vi "PowerSuppliesVoltageControl.vi"(4 "Z+":dbl, 6 "Z-":dbl, 7 "OnOff":bool, 8 "Y+":dbl, 9 "Y-":dbl, 10 "X+":dbl, 11 "X-":dbl) -> (0 "Iz-":dbl)   [LabVIEW 2017]
uses:
  <vilib>/imath/engines/lvmath2/RunTimeEngine/Managers/WorkSpace/UID Generator.vi
  <vilib>/imath/engines/lvmath2/RunTimeEngine/RunTimeType/NIMS_RunTimeType_From StrictType (excl LVString).vi
  <instcachedir>/0/NIMS_RunTimeType_From StrictType (excl LVString)_1019F277F0A747EDBCA0F6C52CA54500.lvgen/NIMS_RunTimeType_From StrictType (excl LVString)_1019F277F0A747EDBCA0F6C52CA54500_000.vi
  <vilib>/imath/engines/lvmath2/RunTimeEngine/LocalVariableDefStatement/MC_LocalVariableDefStatement_Display.vi
  <vilib>/imath/engines/lvmath2/RunTimeEngine/Managers/SymbolTable/Clear UID.vi
  <vilib>/imath/engines/lvmath2/RunTimeEngine/NodeEndStatement/NIMS_NodeEndStatement_Output.vi
  <instcachedir>/0/NIMS_NodeEndStatement_Output_53EC0D466D134D7ABD903AC30B43404B.lvgen/NIMS_NodeEndStatement_Output_53EC0D466D134D7ABD903AC30B43404B_001.vi
  <vilib>/imath/engines/lvmath2/RunTimeEngine/ErrorHandling/NIMS_Finalize Error.vi
  <vilib>/imath/engines/lvmath2/RunTimeEngine/Managers/SymbolTable/NIMS_WorkSpace.lvlib
panel:
  out "Numeric 6":dbl
  out "Numeric 5":dbl
  out "Numeric 4":dbl
  out "Numeric 3":dbl
  out "Numeric 2":dbl
  out "Waveform Chart":dbl(graph)
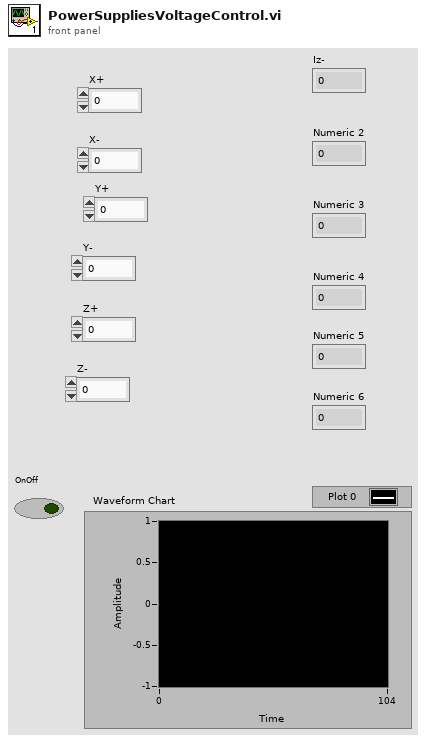
[diagram p1: front panel]
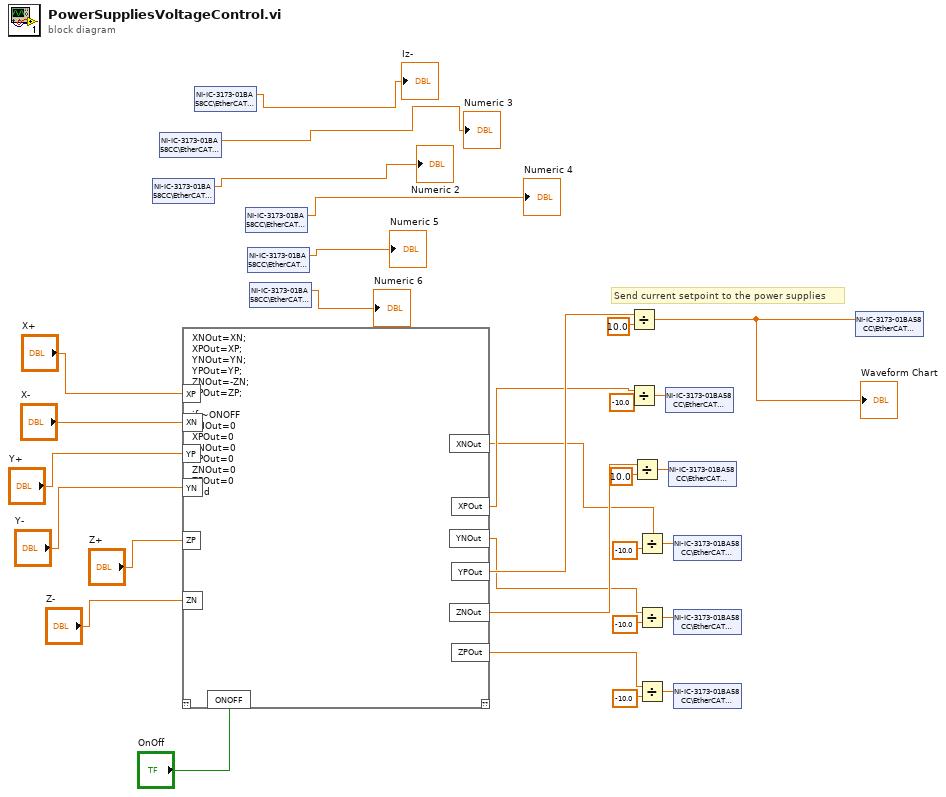
[diagram p0: block diagram]
diagram:
  # "Send current setpoint to the power supplies"
  n1 = shared-variable "NI-IC-3173-01BA58CC\\EtherCAT Master\\Device\\Mod4\\AI2"() -> (→"Numeric 2":dbl)  [unwired: 1 in, 1 out]
  n2 = shared-variable "NI-IC-3173-01BA58CC\\EtherCAT Master\\Device\\Mod4\\AI1"() -> (→"Numeric 3":dbl)  [unwired: 1 in, 1 out]
  n3 = mathscript code="XNOut=XN;\nXPOut=XP;\nYNOut=YN;\nYPOut=YP;\nZNOut=-ZN;\nZPOut=ZP;\n\nif ~ONOFF\nXNOut=0\nXPOut=0\nYNOut=0\nYPOut=0\nZNOut=0\nZPOut=0\nend"("YP"="Y+", "YN"="Y-", "XP"="X+", "XN"="X-", "ZP"="Z+", "ZN"="Z-", "ONOFF"="OnOff") -> ("XNOut"=w11:dbl, "XPOut"=w13:dbl, "YNOut"=w10:dbl, "YPOut"=w14:dbl, "ZNOut"=w12:dbl, "ZPOut"=w9:dbl)  [unwired: 1 in, 1 out]
  n4 = shared-variable "NI-IC-3173-01BA58CC\\EtherCAT Master\\Device\\Mod4\\AI0"() -> (→"Iz-":dbl)  [unwired: 1 in, 1 out]
  n5 = shared-variable "NI-IC-3173-01BA58CC\\EtherCAT Master\\Device\\Mod4\\AI3"() -> (→"Numeric 4":dbl)  [unwired: 1 in, 1 out]
  n6 = shared-variable "NI-IC-3173-01BA58CC\\EtherCAT Master\\Device\\Mod4\\AI4"() -> (→"Numeric 5":dbl)  [unwired: 1 in, 1 out]
  n7 = shared-variable "NI-IC-3173-01BA58CC\\EtherCAT Master\\Device\\Mod4\\AI5"() -> (→"Numeric 6":dbl)  [unwired: 1 in, 1 out]
  n8 = Divide(x=w14, y=10.0) -> (x/y=w8:dbl)
  "Waveform Chart" <- w8
  n9 = Divide(x=w13, y=-10.0) -> (x/y=w25:dbl)
  n10 = Divide(x=w12, y=10.0) -> (x/y=w30:dbl)
  n11 = Divide(x=w11, y=-10.0) -> (x/y=w28:dbl)
  n12 = Divide(x=w10, y=-10.0) -> (x/y=w24:dbl)
  n13 = Divide(x=w9, y=-10.0) -> (x/y=w22:dbl)
  n14 = shared-variable "NI-IC-3173-01BA58CC\\EtherCAT Master\\Device\\Mod1\\AO0"(w25) -> ()  [unwired: 1 in, 1 out]
  n15 = shared-variable "NI-IC-3173-01BA58CC\\EtherCAT Master\\Device\\Mod1\\AO1"(w30) -> ()  [unwired: 1 in, 1 out]
  n16 = shared-variable "NI-IC-3173-01BA58CC\\EtherCAT Master\\Device\\Mod1\\AO3"(w28) -> ()  [unwired: 1 in, 1 out]
  n17 = shared-variable "NI-IC-3173-01BA58CC\\EtherCAT Master\\Device\\Mod1\\AO2"(w24) -> ()  [unwired: 1 in, 1 out]
  n18 = shared-variable "NI-IC-3173-01BA58CC\\EtherCAT Master\\Device\\Mod2\\AO1"(w22) -> ()  [unwired: 1 in, 1 out]
  n19 = shared-variable "NI-IC-3173-01BA58CC\\EtherCAT Master\\Device\\Mod2\\AO0"(w8) -> ()  [unwired: 1 in, 1 out]
